vi "example test.vi"() -> ()   [LabVIEW 2013, in "EthernetIP tests.lvlib"]
uses:
  EthernetIP tests.lvlib
  configuration/EthernetIP configuration.lvclass
  execution/EthernetIP runtime.lvclass
  <vilib>/NI/Tag Bus/tag/Data Type.ctl
  configuration/assembly type.ctl
  <vilib>/NI/Tag Bus/dictionary/data dictionary.lvclass/data dictionary.ctl
  <vilib>/NI/Tag Bus/dictionary/lookup polymorphs/locate U16.vi
  <vilib>/NI/Tag Bus/table/data polymorphs/write one/write U16.vi
  <vilib>/NI/Tag Bus/table/data polymorphs/read one/read U16.vi
  <vilib>/NI/Tag Bus/dictionary/search/find data index.vi
  <vilib>/NI/Tag Bus/dictionary/search/search string list.vi
  <vilib>/NI/Tag Bus/dictionary/tag not found.vi
  <vilib>/NI/Tag Bus/tag/tag descriptor.lvclass
  <vilib>/NI/Tag Bus/dictionary/data dictionary.lvclass
  <vilib>/NI/Tag Bus/table/data table.lvlib
  channel/EthernetIP Channel.lvclass
panel:
  in  "stop":bool
  in  "value TX":u16(slide)=42 scale=0.0..16000.0
  out "value RX":u16(slide) scale=0.0..16000.0
  out "final error":errorcluster
  out "output error":errorcluster
  out "input error":errorcluster
  out "output lookup error":errorcluster
  out "no data written":bool
  out "input lookup error":errorcluster
  out "init error":errorcluster
  out "correct execution settings":bool
  out "serialization problem":errorcluster
  out "invalid configuration":errorcluster
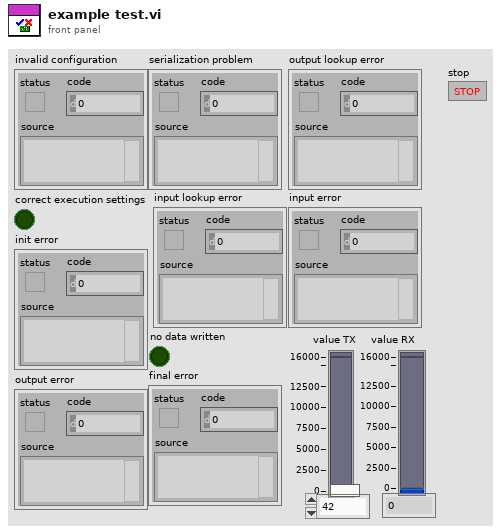
[diagram p1: front panel]
types:
  T1 = typedef "EthernetIP configuration.lvclass/assembly type.ctl" = enum32{"Producing", "Consuming"}
  T2 = typedef "tag bus.lvlib/tag descriptor.lvclass/Data Type.ctl" = enum16{"Double", "Single", "I64", "I32", "I16", "I8", "U64", "U32", "U16", "U8", "Boolean", "String", "Array of Double", "Array of Single", "Array of I64", "Array of I32", "Array of I16", "Array of I8", "Array of U64", "Array of U32", "Array of U16", "Array of U8", "Array of Boolean", "Array of String"}
  T3 = typedef "TBM channel.lvclass/data tables.ctl" = cluster{"input data":T4, "processing parameter":T4, "processing result":T4, "output data":T4}
  T4 = typedef "tag bus.lvlib/dictionary table pair.ctl" = cluster{"data dictionary":refnum<class "data dictionary.lvclass">, "data table":T5}
  T5 = typedef "tag bus.lvlib/data table.lvlib/data table.ctl" = cluster{"Double":dbl[], "Single":sgl[], "I64":i64[], "I32":i32[], "I16":i16[], "I8":i8[], "U64":u64[], "U32":u32[], "U16":u16[], "U8":u8[], "Boolean":bool[], "String":string[], "Array of Double":cluster{"DBL Array":dbl[]}[], "Array of Single":cluster{"SGL Array":sgl[]}[], "Array of I64":cluster{"I64 Array":i64[]}[], "Array of I32":cluster{"I32 Array":i32[]}[], "Array of I16":cluster{"I16 Array":i16[]}[], "Array of I8":cluster{"I8 Array":i8[]}[], "Array of U64":cluster{"U64 Array":u64[]}[], "Array of U32":cluster{"U32 Array":u32[]}[], "Array of U16":cluster{"U16 Array":u16[]}[], "Array of U8":cluster{"U8 Array":u8[]}[], "Array of Boolean":cluster{"Boolean Array":bool[]}[], "Array of String":cluster{"String Array":string[]}[]}
  T6 = typedef "TBM module execution interface.lvclass/execution settings.ctl" = cluster{"reads inputs":bool, "processes data":bool, "writes outputs":bool}
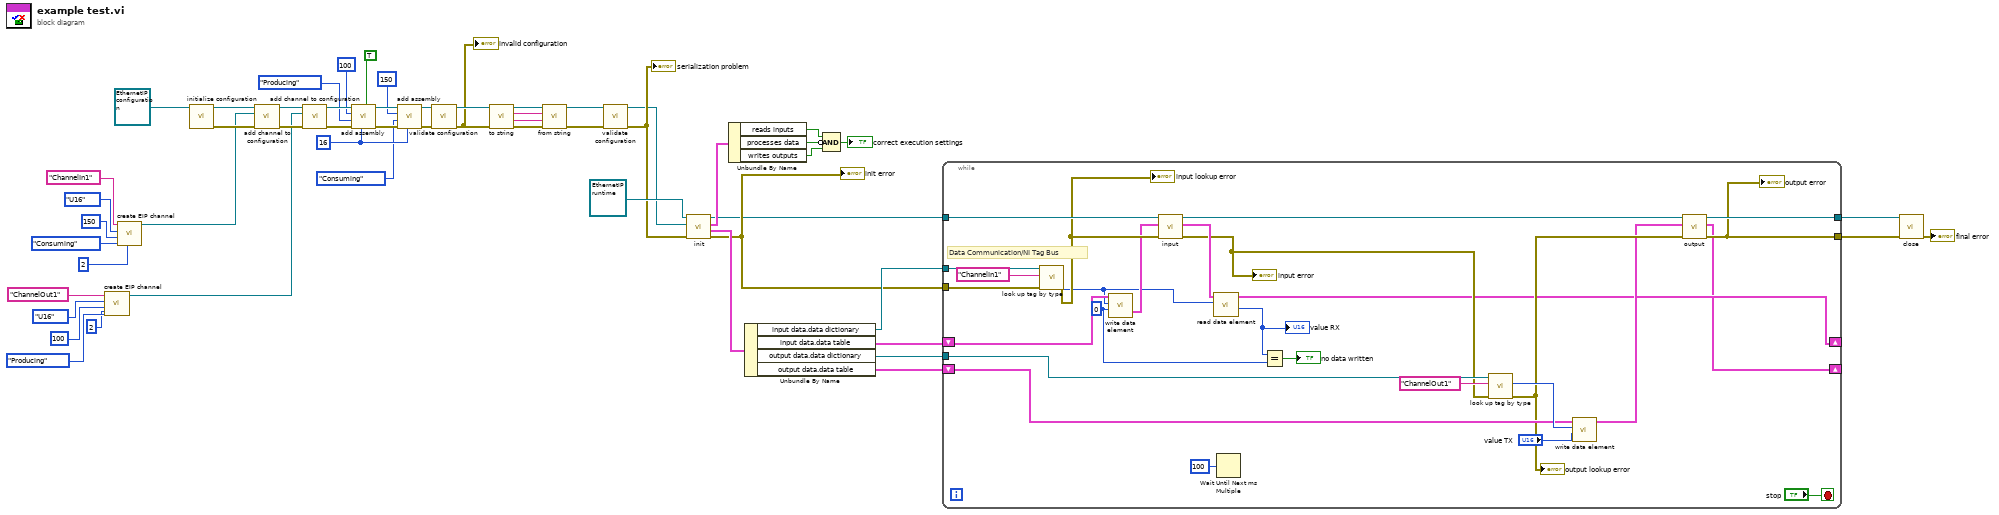
[diagram p0: block diagram]
diagram:
  w6 = u32 16 ("Size (bytes)")
  n1 = call "create EIP channel.vi"("byte index"=2, "Type"=assembly_type."Producing", "Instance ID"=u32 100, "data type"=Data_Type."U16", "name"="ChannelOut1" ("channel name")) -> ("EthernetIP Channel out"=w17:refnum<class "EthernetIP Channel.lvclass">)  [unwired: 6 in]
  n2 = call "create EIP channel.vi"("byte index"=2, "Type"=assembly_type."Consuming", "Instance ID"=u32 150, "data type"=Data_Type."U16", "name"="ChannelIn1" ("channel name")) -> ("EthernetIP Channel out"=w11:refnum<class "EthernetIP Channel.lvclass">)  [unwired: 6 in]
  n3 = call-dynamic "initialize configuration.vi"("configuration in"=refnum<class "EthernetIP configuration.lvclass"> refnum ("tag bus configurable plugin module configuration")) -> ("error out"=w25:errorcluster, "configuration out"=w26:refnum<class "EthernetIP configuration.lvclass">)  [unwired: 8 in, 1 out]
  n4 = call "add channel to configuration.vi"("error in"=w25, "TBM channel in"=w11, "EthernetIP configuration in"=w26) -> ("error out"=w27:errorcluster, "EthernetIP configuration out"=w28:refnum<class "EthernetIP configuration.lvclass">)  [unwired: 7 in]
  n5 = call "add channel to configuration.vi"("error in"=w27, "TBM channel in"=w17, "EthernetIP configuration in"=w28) -> ("error out"=w24:errorcluster, "EthernetIP configuration out"=w9:refnum<class "EthernetIP configuration.lvclass">)  [unwired: 7 in]
  n6 = call "add assembly.vi"("big endian?"=TRUE, "size (bytes)"=w6, "error in"=w24, "Type"=assembly_type."Producing", "instance ID"=u32 100 ("Instance ID"), "EthernetIP configuration in"=w9) -> ("error out"=w10:errorcluster, "EthernetIP configuration out"=w7:refnum<class "EthernetIP configuration.lvclass">)  [unwired: 4 in]
  n7 = call "add assembly.vi"("size (bytes)"=w6, "error in"=w10, "Type"=assembly_type."Consuming", "instance ID"=u32 150 ("Instance ID"), "EthernetIP configuration in"=w7) -> ("error out"=w8:errorcluster, "EthernetIP configuration out"=w23:refnum<class "EthernetIP configuration.lvclass">)  [unwired: 5 in]
  n8 = call-dynamic "validate configuration.vi"("error in"=w8, "EthernetIP configuration in"=w23) -> ("error out"=w54:errorcluster, "EthernetIP configuration out"=w55:refnum<class "EthernetIP configuration.lvclass">)  [unwired: 8 in]
  "invalid configuration" <- w54
  n9 = call-dynamic "to string.vi"("error in"=w54, "EthernetIP configuration in"=w55) -> ("error out"=w50:errorcluster, "data"=w51:string, "version"=w52:string, "EthernetIP configuration out"=w53:refnum<class "EthernetIP configuration.lvclass">)  [unwired: 6 in]
  n10 = call-dynamic "from string.vi"("error in"=w50, "data"=w51, "version"=w52, "EthernetIP configuration in"=w53) -> ("error out"=w48:errorcluster, "EthernetIP configuration out"=w49:refnum<class "EthernetIP configuration.lvclass">)  [unwired: 6 in]
  n11 = call-dynamic "validate configuration.vi"("error in"=w48, "EthernetIP configuration in"=w49) -> ("error out"=w46:errorcluster, "EthernetIP configuration out"=w45:refnum<class "EthernetIP configuration.lvclass">)  [unwired: 8 in]
  "serialization problem" <- w46
  n12 = call-dynamic "init.vi"("error in"=w46, "TBM module configuration in"=w45, "EthernetIP runtime in"=refnum<class "EthernetIP runtime.lvclass"> refnum ("tag bus configurable plugin module")) -> ("error out"=w37:errorcluster, "data allocations"=w39:T3, "execution settings"=w44:T6, "EthernetIP runtime out"=w35:refnum<class "EthernetIP runtime.lvclass">)  [unwired: 5 in]
  "init error" <- w37
  n13 = Unbundle By Name(w44) -> ("reads inputs"=w41:bool, "processes data"=w43:bool, "writes outputs"=w42:bool)
  n14 = Unbundle By Name(w39) -> ("input data.data dictionary"=w38:refnum<class "data dictionary.lvclass">, "input data.data table"=w36:T5, "output data.data dictionary"=w34:refnum<class "data dictionary.lvclass">, "output data.data table"=w33:T5)
  n15 = Compound Arithmetic op=AND(w41, invert w43, w42) -> (→"correct execution settings":bool)
  n16 = while {
    tunnel: w38 -> [w82]
    tunnel: w37 -> [w81]
    tunnel: w35 -> [w78]
    tunnel: w34 -> [w71]
    tunnel: [w62] -> w32
    tunnel: [w61] -> w31
    shift-right: [w58] -> _
    shift-left: w33 -> [w68]
    shift-right: [w59] -> _
    shift-left: w36 -> [w79]
    stop <- "stop" stop-if-true
    w60 = u16 0 ("value")
    # "Data Communication/NI Tag Bus"
    n17 = call-poly <vilib>:"look up tag by type.vi"("error in"=w81, "name"="ChannelIn1" ("channel name"), "data dictionary in"=w82) -> ("error out"=w77:errorcluster, "index"=w74:i32)  [unwired: 6 in, 1 out]
    "input lookup error" <- w77
    n18 = call-poly <vilib>:"write data element.vi"("value"=w60, "index"=w74, "data table in"=w79) -> ("data table out"=w76:T5)  [unwired: 8 in]
    n19 = call-dynamic "input.vi"("error in"=w77, "data table in"=w76, "EthernetIP runtime in"=w78) -> ("error out"=w67:errorcluster, "data table out"=w75:T5, "EthernetIP runtime out"=w64:refnum<class "EthernetIP runtime.lvclass">)  [unwired: 6 in]
    "input error" <- w67
    n20 = call-poly <vilib>:"read data element.vi"("index"=w74, "data table in"=w75) -> ("value"=w73:u16, "data table out"=w59:T5)  [unwired: 8 in]
    "value RX" <- w73
    n21 = Wait Until Next ms Multiple(millisecond multiple=u32 100) -> ()  [unwired: 1 out]
    n22 = Equal?(x=w73, y=w60) -> (x = y?=→"no data written":bool)
    n23 = call-poly <vilib>:"look up tag by type.vi"("error in"=w67, "name"="ChannelOut1" ("channel name"), "data dictionary in"=w71) -> ("error out"=w65:errorcluster, "index"=w69:i32)  [unwired: 6 in, 1 out]
    "output lookup error" <- w65
    n24 = call-poly <vilib>:"write data element.vi"("value"="value TX", "index"=w69, "data table in"=w68) -> ("data table out"=w63:T5)  [unwired: 8 in]
    n25 = call-dynamic "output.vi"("error in"=w65, "data table in"=w63, "EthernetIP runtime in"=w64) -> ("error out"=w61:errorcluster, "data table out"=w58:T5, "EthernetIP runtime out"=w62:refnum<class "EthernetIP runtime.lvclass">)  [unwired: 6 in]
    "output error" <- w61
  }
  n26 = call-dynamic "close.vi"("error in"=w31, "EthernetIP runtime in"=w32) -> ("error out"=→"final error":errorcluster)  [unwired: 9 in]
